vi "_ReadExceldata_EEPROM_vna_jet.vi"(2 "sheet":i32=3, 3 "值列":i32=2, 4 "地址列":i32, 5 "路径":path) -> (0 "Name":string, 1 "EEPROM Map":string[][](array[string]))   [LabVIEW 2011]
panel:
  out "Flag":i32
  out "flag":i32
  out "数据":string[][](array[string])
  in  "Excel._Worksheet":refnum<k7>
  in  "Excel._Application":refnum<k7>
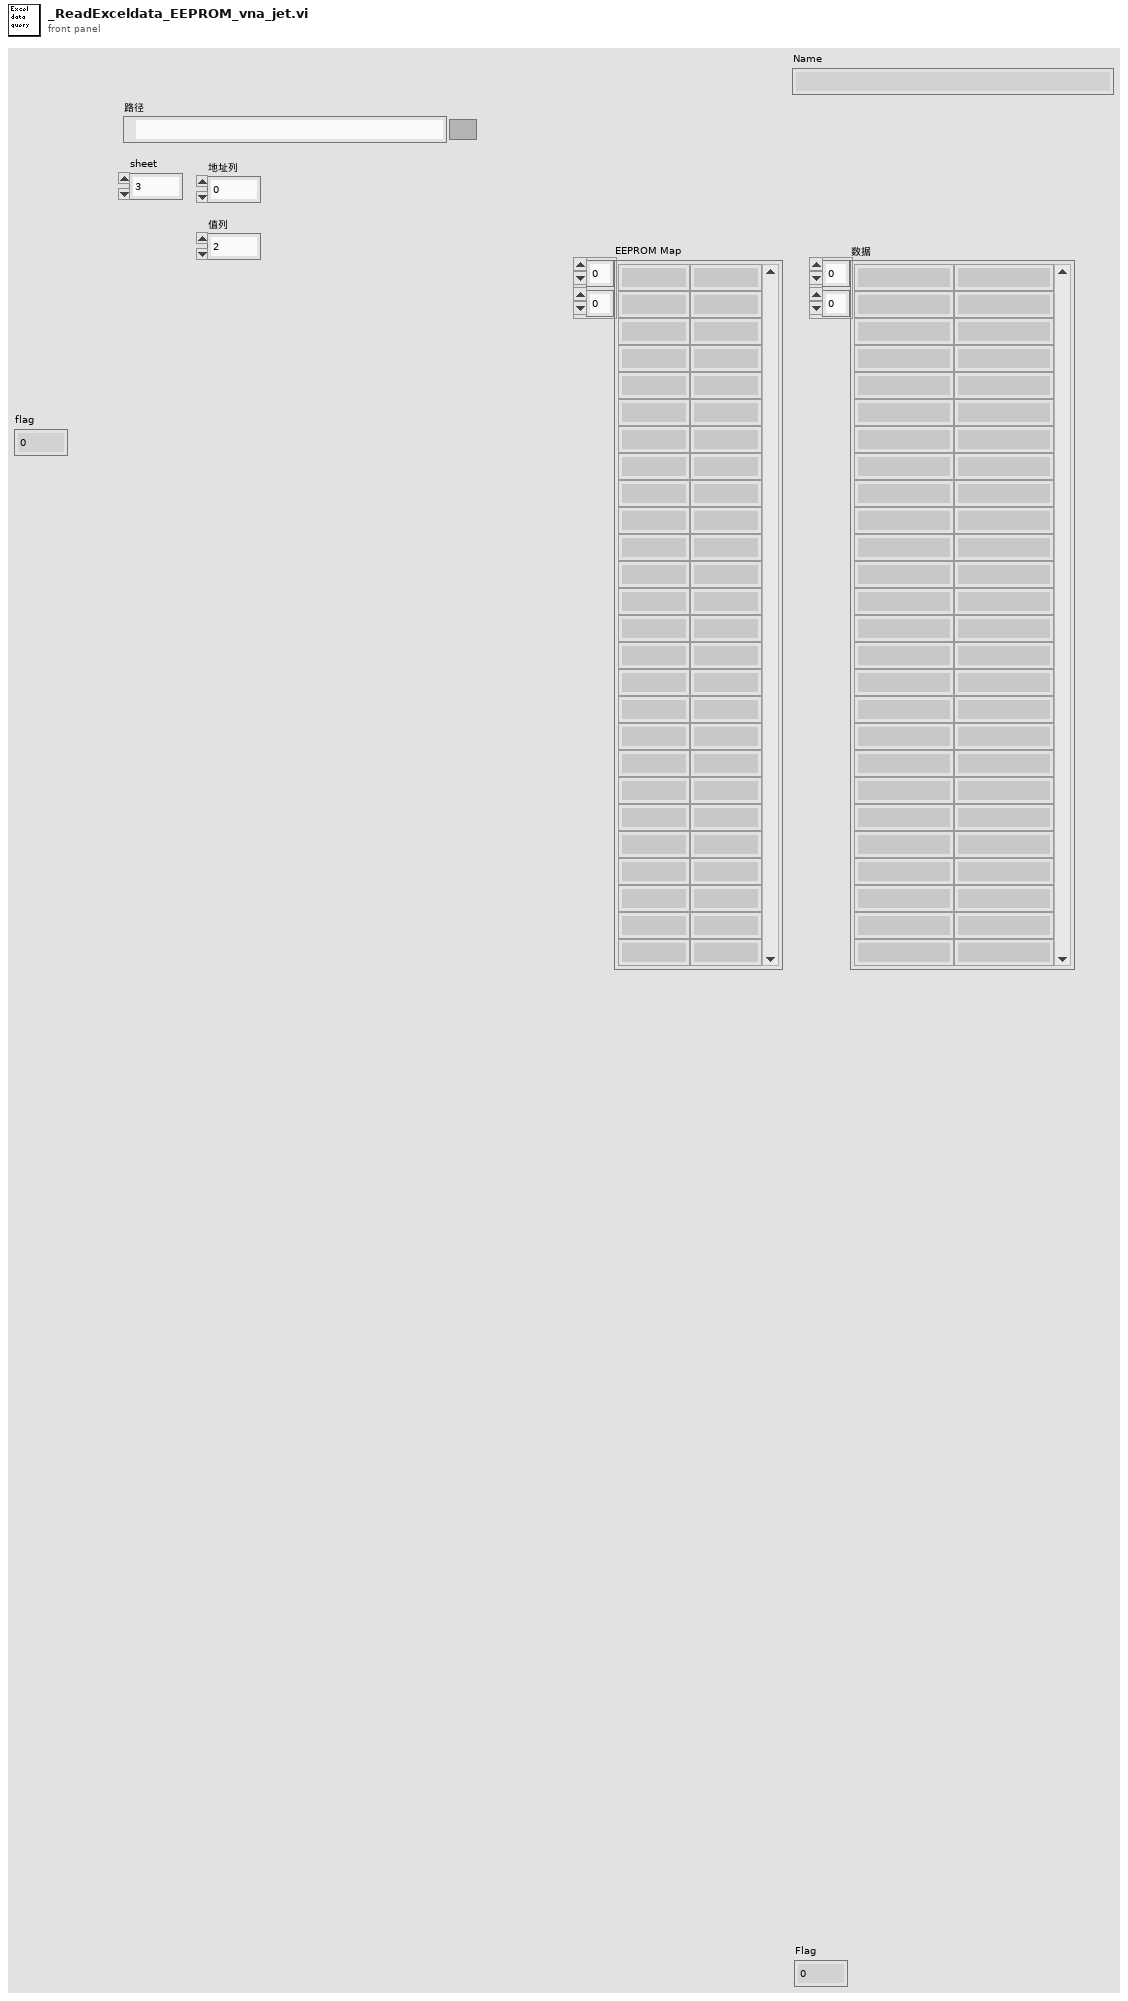
[diagram p1: front panel]
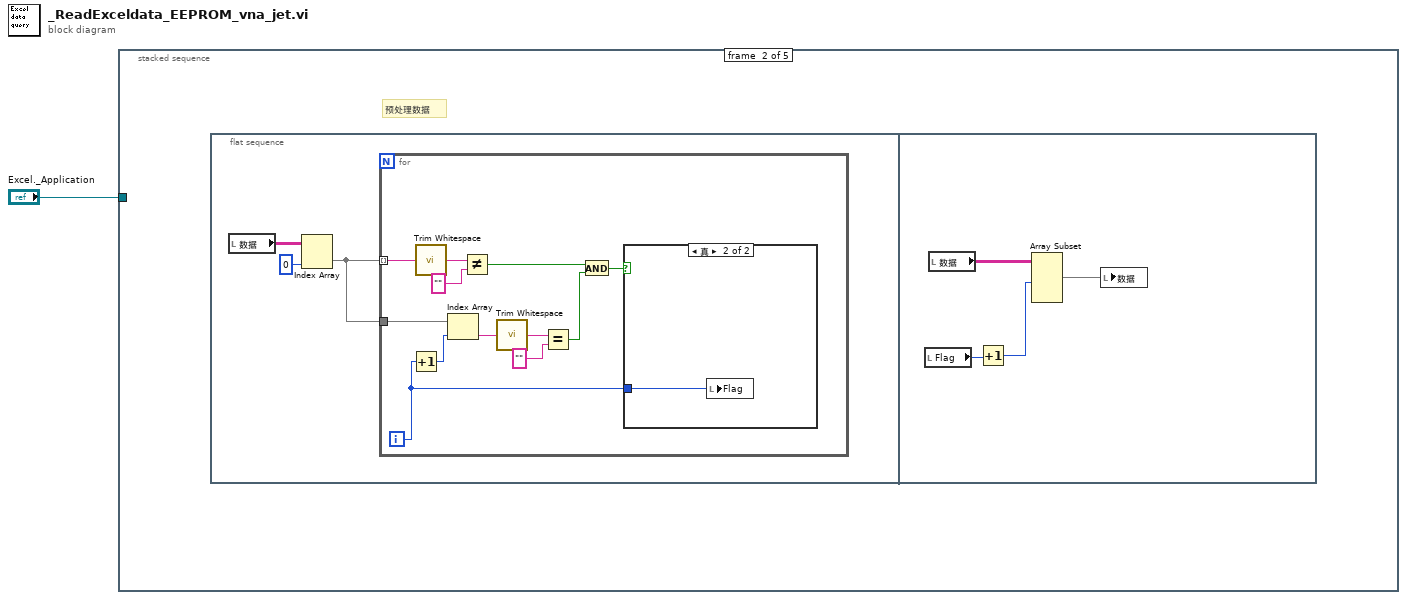
[diagram p0: block diagram]
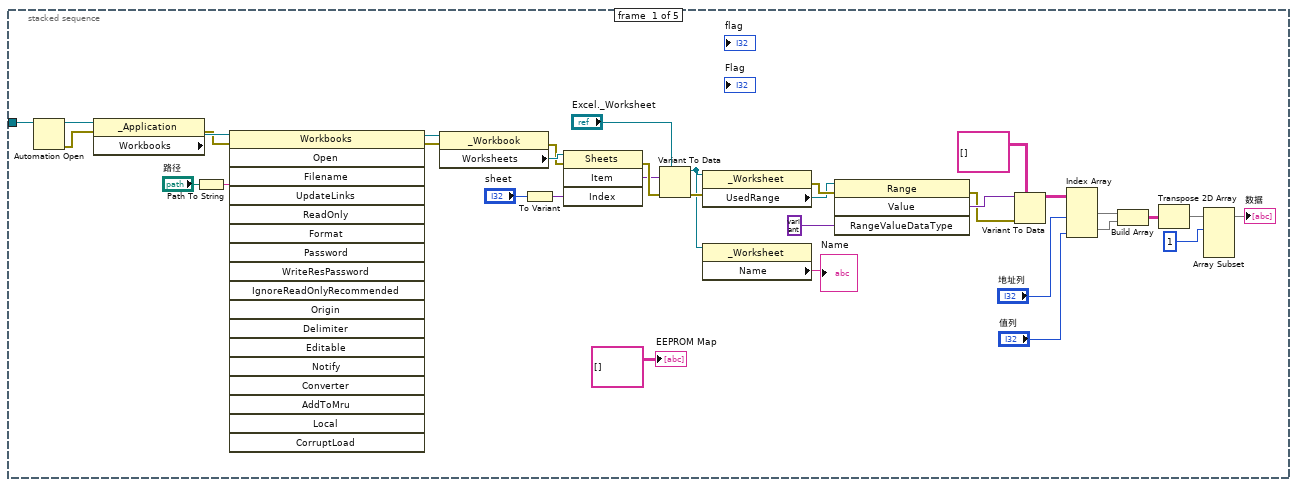
[diagram p2: hidden frame]
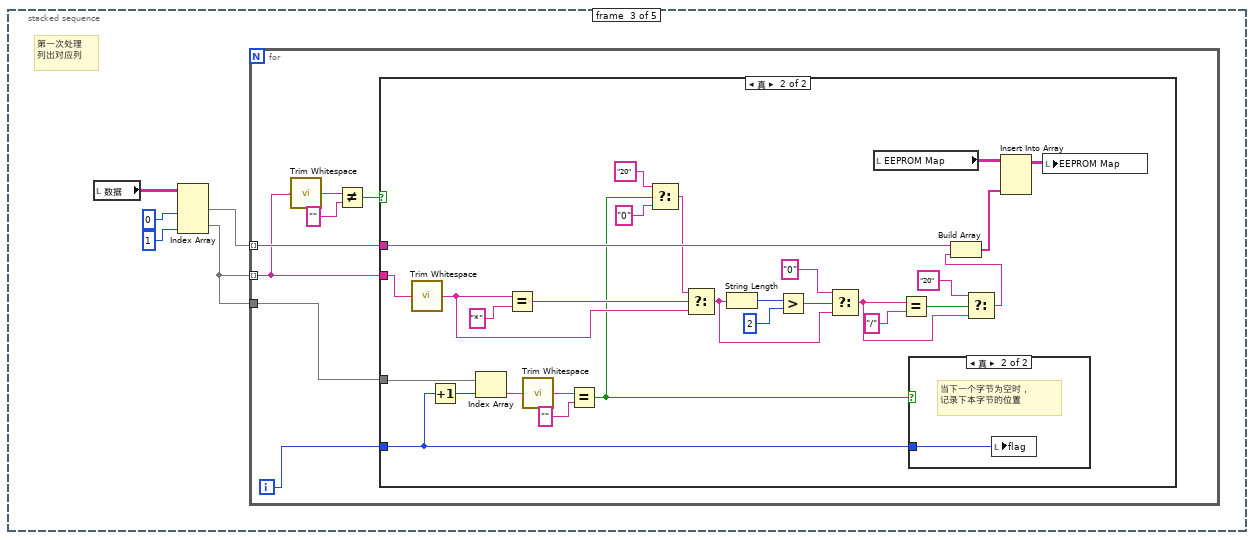
[diagram p4: hidden frame]
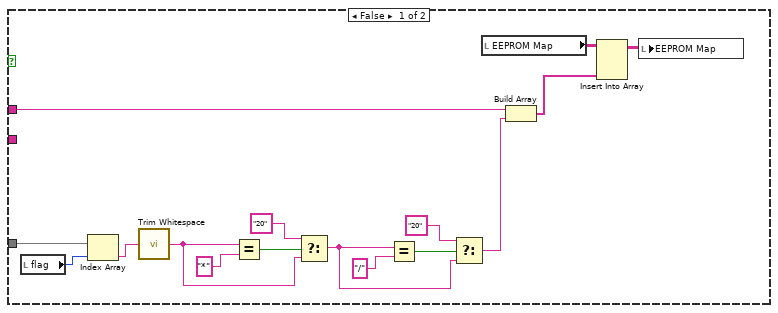
[diagram p5: hidden frame]
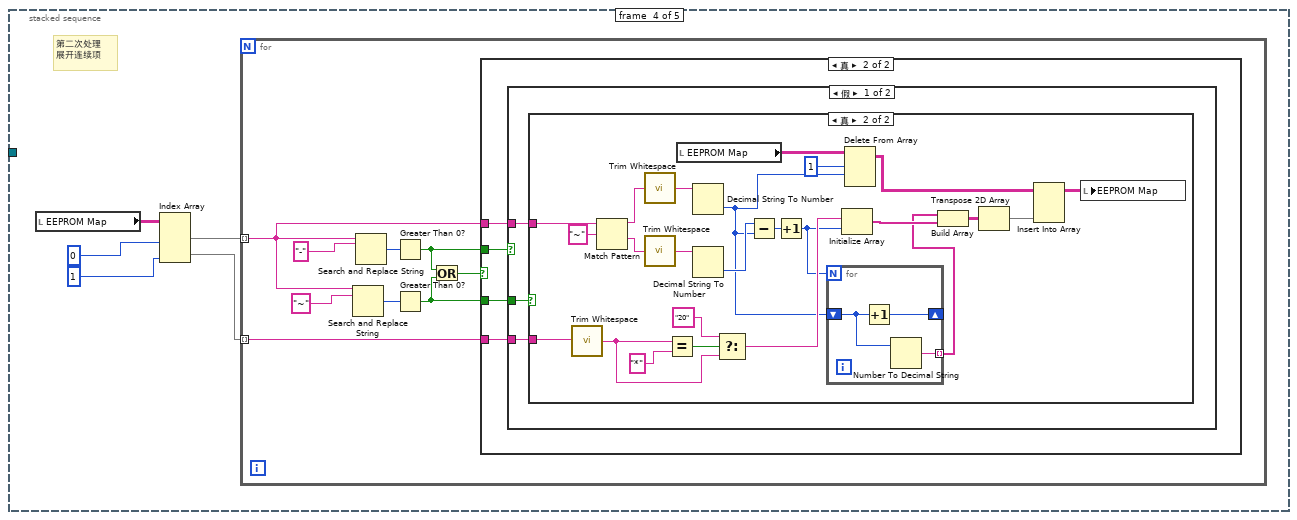
[diagram p7: hidden frame]
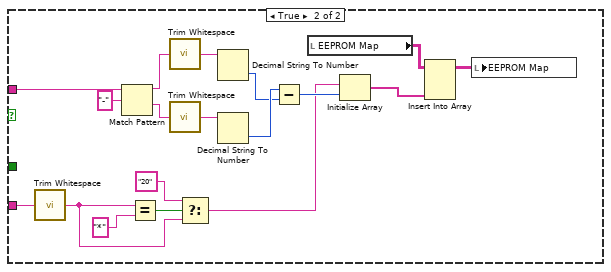
[diagram p10: hidden frame]
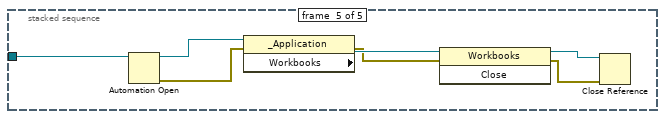
[diagram p11: hidden frame]
diagram:
  n1 = stacked-sequence {
    tunnel: "Excel._Application" -> [w16 _ _ _ w180]
    frame #0 {
      n2 = Automation Open(Automation Refnum=w16) -> (Automation Refnum=w36:refnum<k7>, error out=w35:errorcluster)  [unwired: 3 in]
      n3 = property class="_Application"(reference=w36, error in=w35) -> (error out=w33:errorcluster, "Workbooks"=w34:refnum<k7>)  [unwired: 1 out]
      n4 = Path To String(path="路径") -> (string=w32:string)
      n5 = invoke class="Workbooks" method="Open"(reference=w34, error in=w33, "Filename"=w32) -> (error out=w30:errorcluster, "Open"=w31:refnum<k7>)  [unwired: 15 in, 16 out]
      n6 = property class="_Workbook"(reference=w31, error in=w30) -> (error out=w25:errorcluster, "Worksheets"=w29:refnum<k7>)  [unwired: 1 out]
      n7 = To Variant(anything="sheet") -> (Variant=w27:variant)
      n8 = invoke class="Sheets" method="Item"(reference=w29, error in=w25, "Index"=w27) -> (error out=w26:errorcluster, "Item"=w24:variant)  [unwired: 1 in, 2 out]
      n9 = Variant To Data(error in=w26, type="Excel._Worksheet", Variant=w24) -> (data=w3:refnum<k7>, error out=w22:errorcluster)
      n10 = property class="_Worksheet"(reference=w3, error in=w22) -> (error out=w19:errorcluster, "UsedRange"=w14:refnum<k7>)  [unwired: 1 out]
      n11 = property class="_Worksheet"(reference=w3) -> ("Name"=→"Name":string)  [unwired: 1 in, 2 out]
      n12 = invoke class="Range" method="Value"(reference=w14, error in=w19, "RangeValueDataType"=variant) -> (error out=w17:errorcluster, "Value"=w21:variant)  [unwired: 1 in, 2 out]
      n13 = Variant To Data(error in=w17, type=string[][] [] ("添加的数组"), Variant=w21) -> (data=w12:string[][])  [unwired: 1 out]
      n14 = Index Array(array=w12, index (col) #1="地址列", index (col) #2="值列") -> (element #1=w9:string[], element #2=w8:string[])  [unwired: 2 in]
      n15 = Build Array(w9, w8) -> (w7:string[][])
      n16 = Transpose 2D Array(2D array=w7) -> (transposed array=w5:string[][])
      n17 = Array Subset(array=w5, index (row)=1 ("索引")) -> (→"数据":string[][])  [unwired: 3 in]
      "EEPROM Map" <- string[][] []
    }
    frame #1 {
      # "预处理数据"
      n18 = flat-sequence {
        frame #0 {
          n19 = local read "数据"() -> (w39:string[][])
          n20 = Index Array(array=w39, index (col)=0 ("禁用的索引 (列)")) -> (element=w37:string[])  [unwired: 1 in]
          n21 = for {
            tunnel: w37 -> [w49] mode=indexing
            tunnel: w37 -> [w46]
            i -> [w40]
            n22 = Increment(x=w40) -> (x+1=w45:i32)
            n23 = call <vilib>:"Trim Whitespace.vi"("string"=w49) -> ("trimmed string"=w51:string)  [unwired: 1 in]
            n24 = Index Array(array=w46, index=w45) -> (element=w44:string)
            n25 = Not Equal?(x=w51, y="") -> (x != y?=w43:bool)
            n26 = call <vilib>:"Trim Whitespace.vi"("string"=w44) -> ("trimmed string"=w47:string)  [unwired: 1 in]
            n27 = Equal?(x=w47, y="") -> (x = y?=w42:bool)
            n28 = And(x=w43, y=w42) -> (x .and. y?=w41:bool)
            n29 = case shown="真" w41 {
              tunnel: w40 -> [_ w52]
              frame False {
              }
              frame True {
                n30 = local write "Flag"(w52) -> ()
              }
            }
          }
        }
        frame #1 {
          n31 = local read "Flag"() -> (w55:i32)
          n32 = local read "数据"() -> (w56:string[][])
          n33 = Increment(x=w55) -> (x+1=w54:i32)
          n34 = Array Subset(array=w56, length (row)=w54) -> (w53:string[][])  [unwired: 3 in]
          n35 = local write "数据"(w53) -> ()
        }
      }
    }
    frame #2 {
      # "第一次处理\n列出对应列"
      n36 = local read "数据"() -> (w61:string[][])
      n37 = Index Array(array=w61, index (col) #1=0 ("索引 (列)"), index (col) #2=1 ("索引 (列)")) -> (element #1=w58:string[], element #2=w57:string[])  [unwired: 2 in]
      n38 = for {
        tunnel: w58 -> [w68] mode=indexing
        tunnel: w57 -> [w64] mode=indexing
        tunnel: w57 -> [w62]
        i -> [w63]
        n39 = call <vilib>:"Trim Whitespace.vi"("string"=w64) -> ("trimmed string"=w67:string)  [unwired: 1 in]
        n40 = Not Equal?(x=w67, y="") -> (x != y?=w65:bool)
        n41 = case shown="真" w65 {
          tunnel: w68 -> [w82 w112]
          tunnel: w64 -> [_ w99]
          tunnel: w63 -> [_ w106]
          tunnel: w62 -> [w84 w109]
          frame False {
            n42 = local read "flag"() -> (w83:i32)
            n43 = Index Array(array=w84, index=w83) -> (element=w77:string)
            n44 = call <vilib>:"Trim Whitespace.vi"("string"=w77) -> ("trimmed string"=w75:string)  [unwired: 1 in]
            n45 = Equal?(x=w75, y="*") -> (x = y?=w76:bool)
            n46 = Select(t="20", s=w76, f=w75) -> (s? t:f=w70:string)
            n47 = Equal?(x=w70, y="/") -> (x = y?=w72:bool)
            n48 = Select(t="20", s=w72, f=w70) -> (s? t:f=w69:string)
            n49 = local read "EEPROM Map"() -> (w81:string[][])
            n50 = Build Array(w82, w69) -> (w79:string[])
            n51 = Insert Into Array(array=w81, new element=w79) -> (w80:string[][])  [unwired: 2 in]
            n52 = local write "EEPROM Map"(w80) -> ()
          }
          frame True {
            n53 = call <vilib>:"Trim Whitespace.vi"("string"=w99) -> ("trimmed string"=w100:string)  [unwired: 1 in]
            n54 = Increment(x=w106) -> (x+1=w108:i32)
            n55 = Index Array(array=w109, index=w108) -> (element=w107:string)
            n56 = Equal?(x=w100, y="*") -> (x = y?=w102:bool)
            n57 = call <vilib>:"Trim Whitespace.vi"("string"=w107) -> ("trimmed string"=w110:string)  [unwired: 1 in]
            n58 = Equal?(x=w110, y="") -> (x = y?=w96:bool)
            n59 = Select(t="20", s=w96, f="0") -> (s? t:f=w95:string)
            n60 = Select(t=w95, s=w102, f=w100) -> (s? t:f=w90:string)
            n61 = String Length(string=w90) -> (length=w93:i32)
            n62 = Greater?(x=w93, y=2) -> (0:w94:bool)
            n63 = Select(t="0", s=w94, f=w90) -> (s? t:f=w86:string)
            n64 = local read "EEPROM Map"() -> (w105:string[][])
            n65 = Equal?(x=w86, y="/") -> (x = y?=w88:bool)
            n66 = case shown="真" w96 {
              tunnel: w106 -> [_ w113]
              frame False {
              }
              frame True {
                # "当下一个字节为空时，\n记录下本字节的位置"
                n67 = local write "flag"(w113) -> ()
              }
            }
            n68 = Select(t="20", s=w88, f=w86) -> (s? t:f=w85:string)
            n69 = Build Array(w112, w85) -> (w104:string[])
            n70 = Insert Into Array(array=w105, new element=w104) -> (w103:string[][])  [unwired: 2 in]
            n71 = local write "EEPROM Map"(w103) -> ()
          }
        }
      }
    }
    frame #3 {
      # "第二次处理\n展开连续项"
      n72 = local read "EEPROM Map"() -> (w118:string[][])
      n73 = Index Array(array=w118, index (col) #1=0 ("禁用的索引 (列)"), index (col) #2=1 ("索引 (列)")) -> (element #1=w115:string[], element #2=w114:string[])  [unwired: 2 in]
      n74 = for {
        tunnel: w115 -> [w121] mode=indexing
        tunnel: w114 -> [w120] mode=indexing
        n75 = Search and Replace String(input string=w121, search string="~" ("搜索字符串")) -> (number of replacements=w124:i32)  [unwired: 6 in, 3 out]
        n76 = Search and Replace String(input string=w121, search string="-" ("搜索字符串")) -> (number of replacements=w125:i32)  [unwired: 6 in, 3 out]
        n77 = Greater Than 0?(x=w125) -> (x > 0?=w122:bool)
        n78 = Greater Than 0?(x=w124) -> (x > 0?=w119:bool)
        n79 = Or(x=w122, y=w119) -> (x .or. y?=w123:bool)
        n80 = case shown="真" w123 {
          tunnel: w122 -> [_ w131]
          tunnel: w121 -> [_ w130]
          tunnel: w120 -> [_ w129]
          tunnel: w119 -> [_ w128]
          frame False {
          }
          frame True {
            n81 = case shown="假" w131 {
              tunnel: w130 -> [w133 w179]
              tunnel: w129 -> [w132 w164]
              tunnel: w128 -> [w134 _]
              frame False {
                n82 = case shown="真" w134 {
                  tunnel: w133 -> [_ w152]
                  tunnel: w132 -> [_ w146]
                  frame False {
                  }
                  frame True {
                    n83 = call <vilib>:"Trim Whitespace.vi"("string"=w146) -> ("trimmed string"=w147:string)  [unwired: 1 in]
                    n84 = Match Pattern(string=w152, regular expression="~" ("正则表达式")) -> (before substring=w157:string, after substring=w156:string)  [unwired: 1 in, 2 out]
                    n85 = call <vilib>:"Trim Whitespace.vi"("string"=w157) -> ("trimmed string"=w155:string)  [unwired: 1 in]
                    n86 = call <vilib>:"Trim Whitespace.vi"("string"=w156) -> ("trimmed string"=w154:string)  [unwired: 1 in]
                    n87 = Equal?(x=w147, y="*") -> (x = y?=w150:bool)
                    n88 = local read "EEPROM Map"() -> (w144:string[][])
                    n89 = Decimal String To Number(string=w155) -> (number=w136:i32)  [unwired: 2 in, 1 out]
                    n90 = Decimal String To Number(string=w154) -> (number=w153:i32)  [unwired: 2 in, 1 out]
                    n91 = Select(t="20", s=w150, f=w147) -> (s? t:f=w145:string)
                    n92 = Subtract(x=w153, y=w136) -> (x-y=w141:i32)
                    n93 = Increment(x=w141) -> (x+1=w135:i32)
                    n94 = for {
                      N: w135 -> [_]
                      shift-right: [w161] -> _
                      shift-left: w136 -> [w159]
                      tunnel: [w160] -> w139 mode=indexing
                      n95 = Increment(x=w159) -> (x+1=w161:i32)
                      n96 = Number To Decimal String(number=w159) -> (decimal integer string=w160:string)  [unwired: 1 in]
                    }
                    n97 = Initialize Array(w145, w135) -> (w140:string[])
                    n98 = Delete From Array(array=w144, length=1 ("长度"), index (row)=w136) -> (array with subset deleted=w142:string[][])  [unwired: 1 in, 1 out]
                    n99 = Build Array(w139, w140) -> (w138:string[][])
                    n100 = Transpose 2D Array(2D array=w138) -> (transposed array=w137:string[][])
                    n101 = Insert Into Array(array=w142, new element=w137) -> (w151:string[][])  [unwired: 2 in]
                    n102 = local write "EEPROM Map"(w151) -> ()
                  }
                }
              }
              frame True {
                n103 = call <vilib>:"Trim Whitespace.vi"("string"=w164) -> ("trimmed string"=w163:string)  [unwired: 1 in]
                n104 = Match Pattern(string=w179, regular expression="-" ("正则表达式")) -> (before substring=w177:string, after substring=w176:string)  [unwired: 1 in, 2 out]
                n105 = Equal?(x=w163, y="*") -> (x = y?=w167:bool)
                n106 = call <vilib>:"Trim Whitespace.vi"("string"=w177) -> ("trimmed string"=w175:string)  [unwired: 1 in]
                n107 = call <vilib>:"Trim Whitespace.vi"("string"=w176) -> ("trimmed string"=w174:string)  [unwired: 1 in]
                n108 = Select(t="20", s=w167, f=w163) -> (s? t:f=w162:string)
                n109 = Decimal String To Number(string=w175) -> (number=w172:i32)  [unwired: 2 in, 1 out]
                n110 = Decimal String To Number(string=w174) -> (number=w173:i32)  [unwired: 2 in, 1 out]
                n111 = Subtract(x=w173, y=w172) -> (x-y=w171:i32)
                n112 = local read "EEPROM Map"() -> (w170:string[][])
                n113 = Initialize Array(w162, w171) -> (w168:string[])
                n114 = Insert Into Array(array=w170, new element=w168) -> (w169:string[][])  [unwired: 2 in]
                n115 = local write "EEPROM Map"(w169) -> ()
              }
            }
          }
        }
      }
    }
    frame #4 {
      n116 = Automation Open(Automation Refnum=w180) -> (Automation Refnum=w186:refnum<k7>, error out=w185:errorcluster)  [unwired: 3 in]
      n117 = property class="_Application"(reference=w186, error in=w185) -> (error out=w183:errorcluster, "Workbooks"=w184:refnum<k7>)  [unwired: 1 out]
      n118 = invoke class="Workbooks" method="Close"(reference=w184, error in=w183) -> (reference out=w181:refnum<k7>, error out=w182:errorcluster)  [unwired: 1 in, 1 out]
      n119 = Close Reference(reference=w181, error in (no error)=w182) -> ()  [unwired: 1 out]
    }
  }
